vi "TestKeithley.vi"() -> ()   [LabVIEW 2018]
panel:
  out "error out":errorcluster
  in  "error in (no error)":errorcluster
  out "port out":refnum<visa-resource-name>
  in  "Port":refnum<visa-resource-name>
  out "Current":dbl
  out "Voltage":dbl
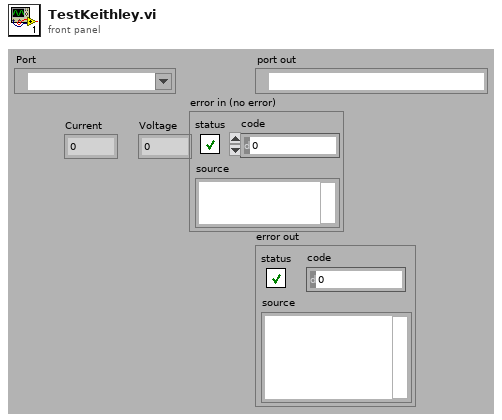
[diagram p1: front panel]
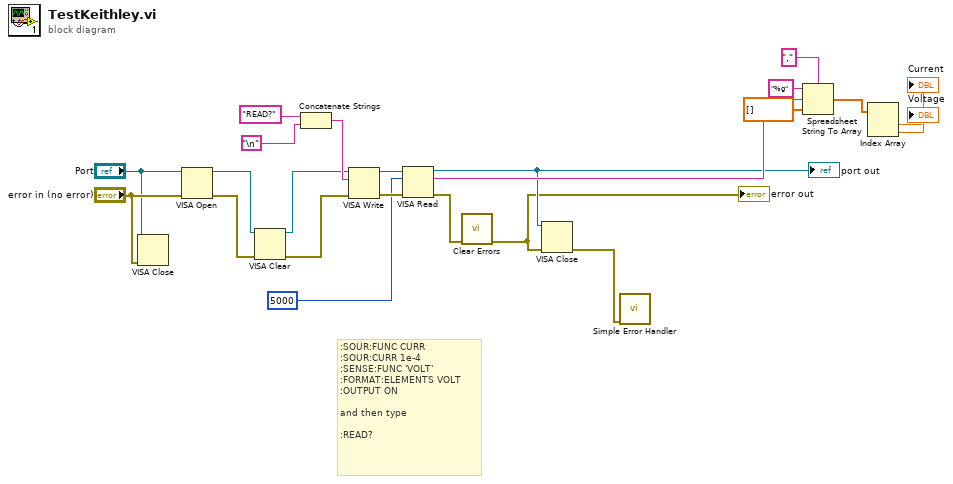
[diagram p0: block diagram]
diagram:
  # ":SOUR:FUNC CURR\n:SOUR:CURR 1e-4\n:SENSE:FUNC 'VOLT'\n:FORMAT:ELEMENTS VOLT\n:OUTPUT ON\n\nand then type\n\n:READ?"
  n1 = VISA Close(VISA resource name="Port", error in (no error)="error in (no error)") -> ()  [unwired: 1 out]
  n2 = VISA Open(error in (no error)="error in (no error)", VISA resource name="Port") -> (VISA resource name=w4:refnum<visa-resource-name>, error out=w2:errorcluster)  [unwired: 3 in]
  n3 = VISA Clear(VISA resource name=w4, error in (no error)=w2) -> (VISA resource name out=w3:refnum<visa-resource-name>, error out=w1:errorcluster)
  n4 = Concatenate Strings("READ?" ("data"), "\n") -> (w15:string)
  n5 = VISA Write(VISA resource name=w3, write buffer=w15, error in (no error)=w1) -> (VISA resource name out=w11:refnum<visa-resource-name>, error out=w16:errorcluster)  [unwired: 1 out]
  n6 = VISA Read(VISA resource name=w11, byte count=5000, error in (no error)=w16) -> (VISA resource name out=w10:refnum<visa-resource-name>, read buffer=w17:string, error out=w9:errorcluster)  [unwired: 1 out]
  "port out" <- w10
  n7 = call <vilib>:"Clear Errors.vi"("error in (no error)"=w9) -> ("error out"=w5:errorcluster)  [unwired: 5 in, 1 out]
  "error out" <- w5
  n8 = VISA Close(VISA resource name=w10, error in (no error)=w5) -> (error out=w6:errorcluster)
  n9 = call <vilib>:"Simple Error Handler.vi"("error in (no error)"=w6) -> ()  [unwired: 4 in, 5 out]
  n10 = Spreadsheet String To Array(delimiter (Tab)=",", format string="%g", spreadsheet string=w17, array type (2D Dbl)=dbl[] []) -> (array=w20:dbl[])
  n11 = Index Array(array=w20) -> (element #1=→"Voltage":dbl, element #2=→"Current":dbl)  [unwired: 2 in]
